vi "Fpga-Convert-Str-to-U64.vi"(10 "startingIndex":i32, 11 "Str.Value":u8[](array[numeric])=[0, 0, 0, 0, 0, 0, 0, 0, 0, 0, 0, 0, 0, 0, 0, 0, 0, 0, 0, 0, 0, 0, 0, 0, 0, 0, 0, 0, 0, 0, 0, 0]) -> (3 "Numeric":u64)   [LabVIEW 2020]
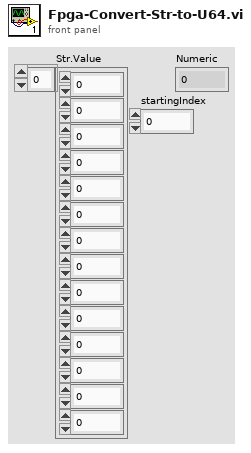
[diagram p1: front panel]
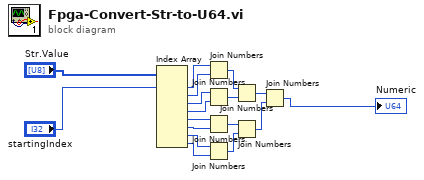
[diagram p0: block diagram]
diagram:
  n1 = Index Array(array="Str.Value", index #1="startingIndex") -> (element #1=w15:u8, element #2=w14:u8, element #3=w13:u8, element #4=w12:u8, element #5=w11:u8, element #6=w10:u8, element #7=w9:u8, element #8=w8:u8)  [unwired: 7 in]
  n2 = Join Numbers(hi=w15, lo=w14) -> ((hi.lo)=w7:u16)
  n3 = Join Numbers(hi=w13, lo=w12) -> ((hi.lo)=w6:u16)
  n4 = Join Numbers(hi=w11, lo=w10) -> ((hi.lo)=w5:u16)
  n5 = Join Numbers(hi=w9, lo=w8) -> ((hi.lo)=w4:u16)
  n6 = Join Numbers(hi=w7, lo=w6) -> ((hi.lo)=w2:u32)
  n7 = Join Numbers(hi=w5, lo=w4) -> ((hi.lo)=w3:u32)
  n8 = Join Numbers(hi=w2, lo=w3) -> ((hi.lo)=→"Numeric":u64)
